vi "ReportHead_A131258.vi"(8 "error in (no error)":errorcluster caption="错误输入（无错误）", 11 "产品状态":string) -> (0 "error out":errorcluster caption="错误输出", 3 "report out":refnum<class "NI_report.lvclass"> caption="报表输出")   [LabVIEW 2018]
uses:
  <vilib>/Utility/NIReport.llb/NI_report.lvclass
  <vilib>/addons/_office/_exclsub.llb/font.ctl
  Database/Global1.vi
  <vilib>/addons/_office/NI_ReportGenerationToolkit.lvlib
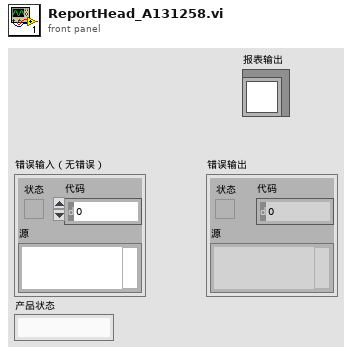
[diagram p1: front panel]
types:
  T1 = cluster{"操作者编号":string, "操作者姓名":string, "操作者权限":string, "联机状态":string, "产品型号":string, "产品状态":string}
  T2 = cluster{"top":dbl, "left":dbl, "right":dbl, "bottom":dbl}
  T3 = cluster{"Charset (-1)":i16, "Weight (-1)":i16, "Name":string, "Size":string}
  T4 = cluster{"Italic":enum16{"Italic Unchanged", "Italic On", "Italic Off"}, "Strike Through":enum16{"Strike Through Unchanged", "Strike Through On", "Strike Through Off"}, "Underline":enum16{"Underline Unchanged", "Underline On", "Underline Off"}, "Bold":enum16{"Bold Unchanged", "Bold On", "Bold Off"}}
  T5 = typedef "NI_ReportGenerationToolkit.lvlib/font.ctl" = cluster{"font name":string, "font size":dbl, "bold":u16, "italic":u16, "underline":u16, "strike through":u16, "font color":u32}
  T6 = enum16{"maximized", "minimized", "normal", "no change"}
  T7 = enum16{"Standard Report", "HTML", "Word", "Excel"}
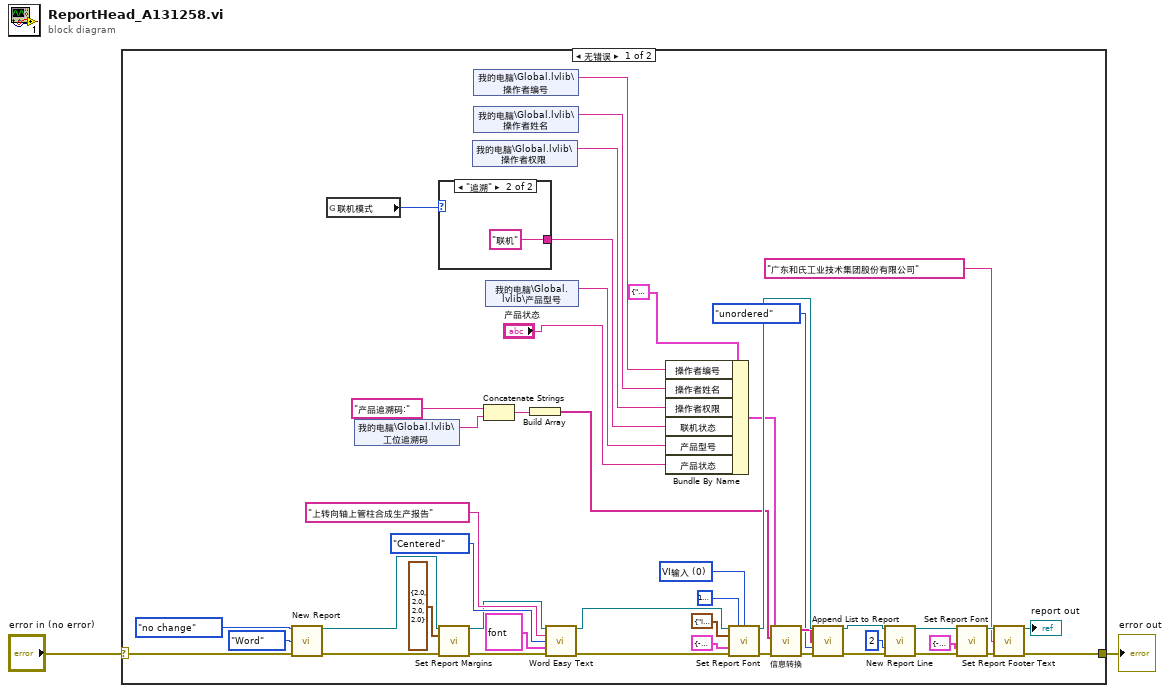
[diagram p0: block diagram]
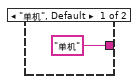
[diagram p2: hidden frame]
diagram:
  n1 = case shown="无错误" "error in (no error)" {
    selector: "error in (no error)" -> [w21 w51]
    tunnel: [w17 w51] -> w1
    frame No Error {
      w41 = u16 0 items=["VI输入", "字体对话框"] ("font settings source")
      n2 = call <vilib>:"New Report.vi"("window state (normal)"=T6."no change", "report type"=T7."Word", "error in (no error)"=w21) -> ("report out"=w34:refnum<class "NI_report.lvclass">, "error out"=w31:errorcluster)  [unwired: 11 in]
      n3 = global read "Global1.vi" "联机模式"() -> (w3:enum16{"单机", "追溯"})
      n4 = shared-variable "我的电脑\\Global.lvlib\\工位追溯码"() -> (w7:string)  [unwired: 1 in, 1 out]
      n5 = case shown="\"追溯\"" w3 {
        tunnel: ["单机" "联机"] -> w11
        frame "单机", Default {
        }
        frame "追溯" {
        }
      }
      n6 = call-dynamic "Set Report Margins.vi"("report in"=w34, "margins (1.00)"=T2 {"top"=2.0, "left"=2.0, "right"=2.0, "bottom"=2.0}, "error in (no error)"=w31) -> ("report out"=w33:refnum<class "NI_report.lvclass">, "error out"=w32:errorcluster)  [unwired: 10 in, 1 out]
      n7 = shared-variable "我的电脑\\Global.lvlib\\操作者权限"() -> (w14:string)  [unwired: 1 in, 1 out]
      n8 = shared-variable "我的电脑\\Global.lvlib\\操作者编号"() -> (w15:string)  [unwired: 1 in, 1 out]
      n9 = shared-variable "我的电脑\\Global.lvlib\\操作者姓名"() -> (w13:string)  [unwired: 1 in, 1 out]
      n10 = Concatenate Strings("产品追溯码:", w7) -> (w6:string)
      n11 = shared-variable "我的电脑\\Global.lvlib\\产品型号"() -> (w12:string)  [unwired: 1 in, 1 out]
      n12 = Build Array(w6) -> (w5:string[])
      n13 = call <vilib>:"Word Easy Text.vi"("report in"=w33, "text"="上转向轴上管柱合成生产报告", "alignment (left)"=enum16{"Left", "Centered", "Right", "Justify"}."Centered", "font"=T5 {"font name"="楷体", "font size"=26.0, "bold"=1, "italic"=2, "underline"=2, "strike through"=2, "font color"=16777228}, "error in (no error)"=w32) -> ("report out"=w43:refnum<class "NI_report.lvclass">, "error out"=w42:errorcluster)  [unwired: 8 in, 1 out]
      n14 = Bundle By Name(cluster=T1 {"操作者编号"="001", "操作者姓名"="Administrator", "操作者权限"="系统管理员", "联机状态"="单机", "产品型号"="SL7202", "产品状态"=""} ("测试信息"), "操作者编号"=w15, "操作者姓名"=w13, "操作者权限"=w14, "联机状态"=w11, "产品型号"=w12, "产品状态"="产品状态") -> (w9:T1)
      n15 = call-dynamic "Set Report Font.vi"("report in"=w43, "text color (unchanged)"=u32 16777224, "font settings source (VI Inputs)"=w41, "text options"=T4 {"Italic"=enum."Italic Off", "Strike Through"=enum."Strike Through Unchanged", "Underline"=enum."Underline Off", "Bold"=enum."Bold Off"}, "font settings"=T3 {"Charset (-1)"=-1, "Weight (-1)"=-1, "Name"="微软雅黑 Light", "Size"="12 "}, "error in (no error)"=w42) -> ("report out"=w29:refnum<class "NI_report.lvclass">, "error out"=w20:errorcluster)  [unwired: 7 in, 1 out]
      n16 = call "信息转换.vi"("错误输入（无错误）"=w20, "追溯码"=w5, "测试信息"=w9) -> ("错误输出"=w19:errorcluster, "信息输出"=w22:string[])  [unwired: 7 in]
      n17 = call-dynamic "Append List to Report.vi"("report in"=w29, "list elements"=w22, "list type (ordered)"=enum16{"unordered", "ordered"}."unordered", "error in (no error)"=w19) -> ("report out"=w24:refnum<class "NI_report.lvclass">, "error out"=w23:errorcluster)  [unwired: 8 in, 2 out]
      n18 = call-dynamic "New Report Line.vi"("report in"=w24, "number of lines (1)"=2, "error in (no error)"=w23) -> ("report out"=w27:refnum<class "NI_report.lvclass">, "error out"=w28:errorcluster)  [unwired: 11 in]
      n19 = call-dynamic "Set Report Font.vi"("report in"=w27, "font settings"=T3 {"Charset (-1)"=-1, "Weight (-1)"=-1, "Name"="楷体", "Size"="9 "}, "error in (no error)"=w28) -> ("report out"=w38:refnum<class "NI_report.lvclass">, "error out"=w37:errorcluster)  [unwired: 10 in, 1 out]
      n20 = call-dynamic "Set Report Footer Text.vi"("report in"=w38, "center footer text"="广东和氏工业技术集团股份有限公司", "error in (no error)"=w37) -> ("report out"=→"report out":refnum<class "NI_report.lvclass">, "error out"=w17:errorcluster)  [unwired: 11 in]
    }
    frame Error {
    }
  }
  "error out" <- w1
